vi "Do API Request.vi"(6 "timeout (30000)":i32=30000, 7 "Method (Auto, see Payload)":T1, 8 "error in (no error)":errorcluster, 9 "Payload (Empty = GET, payload = POST)":string, 10 "API Endpoint":T2=enum."packages/search", 11 "GCentral API in":refnum<class "GCentral API.lvclass">) -> (0 "error out":errorcluster, 1 "Response":string, 2 "Headers":map{string, string}(c390), 3 "GCentral API out":refnum<class "GCentral API.lvclass">, 4 "Debug Link":string)   [LabVIEW 2020, in "GCentral-API.lvlib" / "GCentral API.lvclass"]
uses:
  GCentral API.lvclass
  API Endpoint.ctl
  Method.ctl
  <vilib>/httpClient/POSTBuffer.vi
  <vilib>/httpClient/LabVIEWHTTPClient.lvlib
  GCentral-API.lvlib
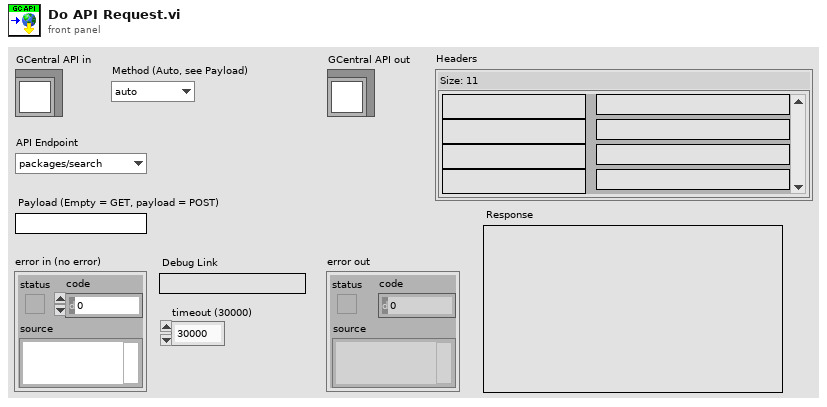
[diagram p1: front panel]
types:
  T1 = typedef "GCentral-API.lvlib/Method.ctl" = enum16{"auto", "GET", "POST"}
  T2 = typedef "GCentral-API.lvlib/API Endpoint.ctl" = enum16{"packages/list", "packages/search"}
  T3 = typedef "LabVIEWHTTPClient.lvlib/ClientHandle.ctl" = refnum<k1>
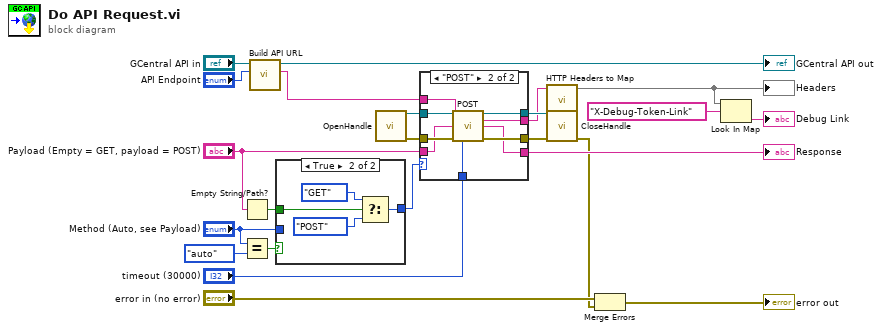
[diagram p0: block diagram]
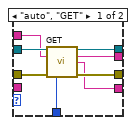
[diagram p3: hidden frame]
diagram:
  n1 = Empty String/Path?(string/path="Payload (Empty = GET, payload = POST)") -> (empty?=w16:bool)
  n2 = Equal?(x="Method (Auto, see Payload)", y=Method."auto") -> (x = y?=w18:bool)
  n3 = call "Build API URL.vi"("API Endpoint"="API Endpoint", "GCentral API in"="GCentral API in") -> ("URL"=w14:string, "GCentral API out"=→"GCentral API out":refnum<class "GCentral API.lvclass">)  [unwired: 7 in, 1 out]
  n4 = case shown="True" w18 {
    tunnel: "Method (Auto, see Payload)" -> [w24 _]
    tunnel: w16 -> [_ w28]
    tunnel: [w24 w25] -> w15
    frame False {
    }
    frame True {
      n5 = Select(t=Method."GET" ("y"), s=w28, f=Method."POST" ("y")) -> (s? t:f=w25:T1)
    }
  }
  n6 = call <vilib>:"OpenHandle.vi"() -> ("client handle out"=w21:T3, "error out"=w20:errorcluster)  [unwired: 14 in]
  n7 = case shown="\"POST\"" w15 {
    tunnel: w21 -> [w35 w45]
    tunnel: w20 -> [w36 w44]
    tunnel: [w33 w43] -> w10
    tunnel: [w34 w42] -> w11
    tunnel: w14 -> [w32 w41]
    tunnel: "timeout (30000)" -> [w31 w40]
    tunnel: "Payload (Empty = GET, payload = POST)" -> [_ w39]
    tunnel: [w30 w37] -> w4
    tunnel: [w29 w38] -> w9
    frame "auto", "GET" {
      n8 = call <vilib>:"GET.vi"("client handle"=w35, "url"=w32, "error in (no error)"=w36, "timeout (10000)"=w31) -> ("client handle out"=w34:T3, "headers"=w30:string, "body"=w29:string, "error out"=w33:errorcluster)  [unwired: 8 in]
    }
    frame "POST" {
      n9 = call-poly <vilib>:"POST.vi"("client handle"=w45, "url"=w41, "buffer"=w39, "error in (no error)"=w44, "timeout (10000)"=w40) -> ("client handle out"=w42:T3, "headers"=w37:string, "body"=w38:string, "error out"=w43:errorcluster)  [unwired: 7 in]
    }
  }
  "Response" <- w9
  n10 = call "HTTP Headers to Map.vi"("Headers"=w4) -> ("Map"=w3:map{string, string})  [unwired: 10 in]
  "Headers" <- w3
  n11 = call <vilib>:"CloseHandle.vi"("client handle"=w11, "error in (no error)"=w10) -> ("error out"=w7:errorcluster)  [unwired: 13 in]
  n12 = Merge Errors("error in (no error)", w7) -> (→"error out":errorcluster)
  n13 = Look In Map(map=w3, key="X-Debug-Token-Link") -> (value=→"Debug Link":string)  [unwired: 1 in, 1 out]
